vi "Vizualise Filter.vi"(10 "Reference Signal":waveform(dbl), 11 "CtlRef":refnum<vi>) -> (0 "Order":i32, 1 "Fc Low":dbl, 2 "Fc High":dbl, 3 "Type":T1, 4 "Filter Magnitude":cluster{"f0":dbl, "df":dbl, "magnitude":dbl[]}(graph))   [LabVIEW 2014]
uses:
  <vilib>/Analysis/3filter.llb/Filter Passband Type.ctl
  <vilib>/Utility/miscctls.llb/LVOutOfRangeActionTypeDef.ctl
  <vilib>/Analysis/3filter.llb/Butterworth Filter (DBL).vi
  <vilib>/express/express analysis/Spectral/Block/exnSpectralBlock spectral measurements peak poly.vi
  <vilib>/express/express analysis/Spectral/Block/exnSpectralBlock spectral measurements peak WFM.vi
  <vilib>/express/express analysis/Spectral/XNode/ExpressSpectralMeasurementsBlockNode.xnode
  <vilib>/Analysis/NI_AALBase.lvlib
  <vilib>/measure/NI_MABase.lvlib
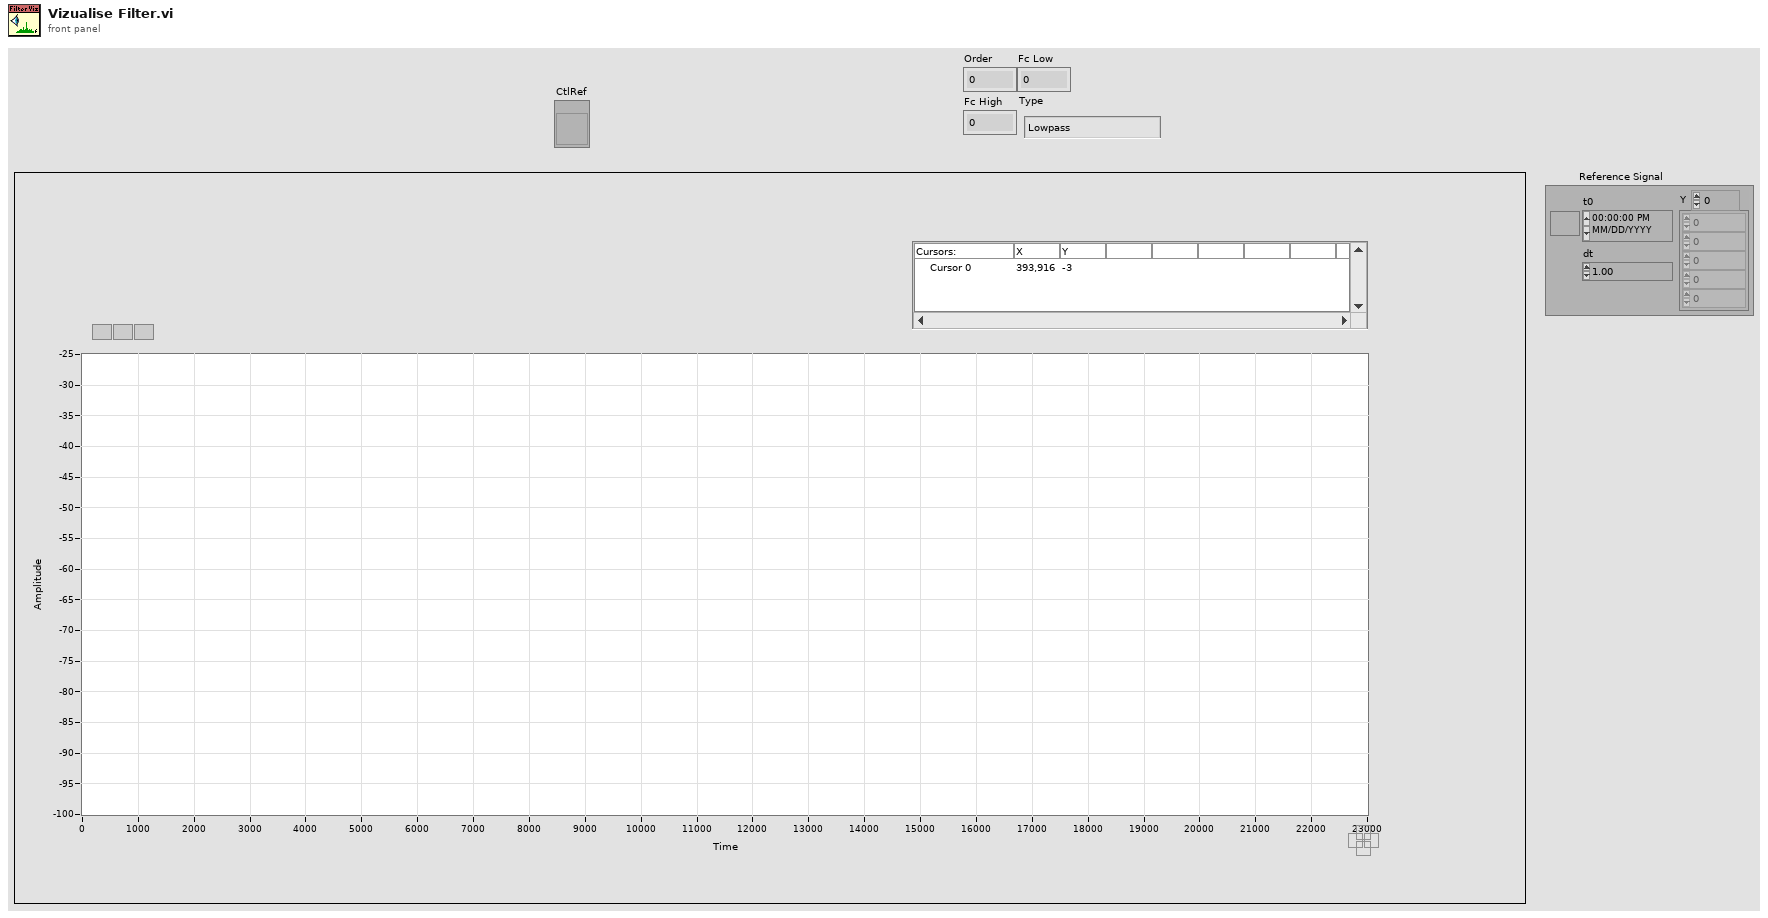
[diagram p1: front panel]
types:
  T1 = typedef "NI_AALBase.lvlib/Filter Passband Type.ctl" = enum32{"Lowpass", "Highpass", "Bandpass", "Bandstop"}
  T2 = typedef "LVOutOfRangeActionTypeDef.ctl" = cluster{"Out of Range Action Minimum":u8, "Out of Range Action Maximum":u8, "Out of Range Action Increment":u8}
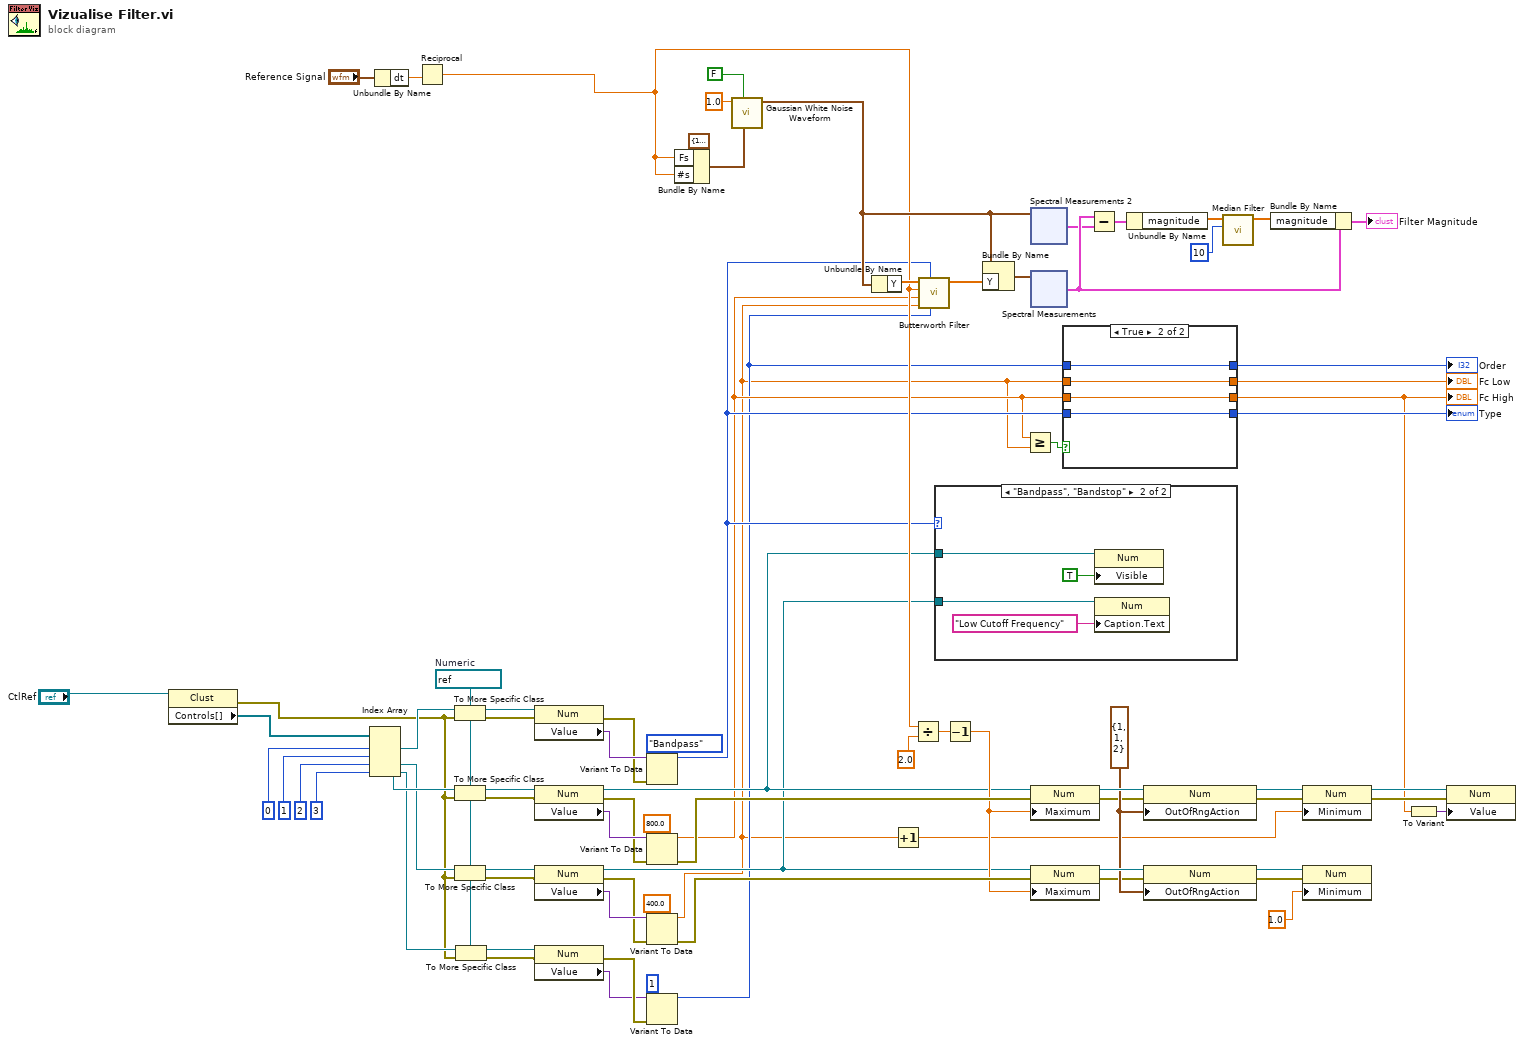
[diagram p0: block diagram]
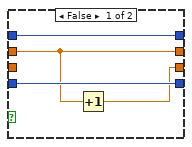
[diagram p2: hidden frame]
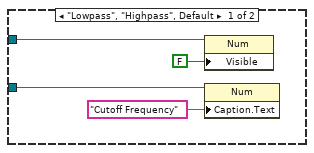
[diagram p3: hidden frame]
diagram:
  w46 = T2 {"Out of Range Action Minimum"=1, "Out of Range Action Maximum"=1, "Out of Range Action Increment"=2} ("Response to Value Outside Limits")
  w51 = refnum<vi> refnum  # Numeric
  n1 = property class="Clust"(reference="CtlRef") -> (error out=w24:errorcluster, "Controls[]"=w65:refnum<vi>[])  [unwired: 1 in, 1 out]
  n2 = Index Array(array=w65, index #1=0 ("index"), index #2=1 ("index"), index #3=2 ("index"), index #4=3 ("index")) -> (element #1=w60:refnum<vi>, element #2=w59:refnum<vi>, element #3=w58:refnum<vi>, element #4=w57:refnum<vi>)
  n3 = Unbundle By Name("Reference Signal") -> ("dt"=w17:dbl)
  n4 = Reciprocal(x=w17) -> (1/x=w16:dbl)
  n5 = To More Specific Class(target class=w51, reference=w60, error in=w24) -> (specific class reference=w56:refnum<vi>, error out=w55:errorcluster)
  n6 = To More Specific Class(target class=w51, reference=w59, error in=w24) -> (specific class reference=w34:refnum<vi>, error out=w35:errorcluster)
  n7 = To More Specific Class(target class=w51, reference=w58, error in=w24) -> (specific class reference=w33:refnum<vi>, error out=w36:errorcluster)
  n8 = To More Specific Class(target class=w51, reference=w57, error in=w24) -> (specific class reference=w32:refnum<vi>, error out=w37:errorcluster)
  n9 = property class="Num"(reference=w56, error in=w55) -> (error out=w53:errorcluster, "Value"=w54:variant)  [unwired: 1 out]
  n10 = property class="Num"(reference=w34, error in=w35) -> (reference out=w15:refnum<vi>, error out=w28:errorcluster, "Value"=w41:variant)
  n11 = property class="Num"(reference=w33, error in=w36) -> (reference out=w14:refnum<vi>, error out=w27:errorcluster, "Value"=w40:variant)
  n12 = property class="Num"(reference=w32, error in=w37) -> (error out=w39:errorcluster, "Value"=w38:variant)  [unwired: 1 out]
  n13 = Variant To Data(error in=w53, type=Filter_Passband_Type."Bandpass" ("filter type"), Variant=w54) -> (data=w11:T1)  [unwired: 1 out]
  n14 = Variant To Data(error in=w28, type=800.0 ("high cutoff freq"), Variant=w41) -> (data=w10:dbl, error out=w25:errorcluster)
  n15 = Variant To Data(error in=w27, type=400.0 ("low cutoff freq"), Variant=w40) -> (data=w1:dbl, error out=w26:errorcluster)
  n16 = Variant To Data(error in=w39, type=1 ("order"), Variant=w38) -> (data=w9:i32)  [unwired: 1 out]
  n17 = Bundle By Name(cluster=cluster{"Fs":dbl, "#s":dbl} {"Fs"=10000.0, "#s"=10000.0} ("sampling info"), "Fs"=w16, "#s"=w16) -> (w76:cluster{"Fs":dbl, "#s":dbl})
  n18 = call <vilib>:"Gaussian White Noise Waveform.vi"("sampling info"=w76, "reset signal"=FALSE, "standard deviation"=1.0 ("amplitude")) -> ("signal out"=w23:waveform(dbl))  [unwired: 7 in, 1 out]
  n19 = Unbundle By Name(w23) -> ("Y"=w78:dbl[])
  n20 = Increment(x=w1) -> (x+1=w13:dbl)
  n21 = Divide(x=w16, y=2.0) -> (x/y=w22:dbl)
  n22 = call-poly <vilib>:"Butterworth Filter.vi"("order"=w9, "filter type"=w11, "low cutoff freq: fl"=w1, "high cutoff freq: fh"=w10, "sampling freq: fs"=w16, "X"=w78) -> ("Filtered X"=w80:dbl[])  [unwired: 2 in, 1 out]
  n23 = case shown="\"Bandpass\", \"Bandstop\"" w11 {
    tunnel: w15 -> [w82 w86]
    tunnel: w14 -> [w81 w85]
    frame "Lowpass", "Highpass", Default {
      n24 = property class="Num"(reference=w82, "Visible"=FALSE) -> ()  [unwired: 1 in, 2 out]
      n25 = property class="Num"(reference=w81, "Caption.Text"="Cutoff Frequency") -> ()  [unwired: 1 in, 2 out]
    }
    frame "Bandpass", "Bandstop" {
      n26 = property class="Num"(reference=w86, "Visible"=TRUE) -> ()  [unwired: 1 in, 2 out]
      n27 = property class="Num"(reference=w85, "Caption.Text"="Low Cutoff Frequency") -> ()  [unwired: 1 in, 2 out]
    }
  }
  n28 = Decrement(x=w22) -> (x-1=w20:dbl)
  n29 = Bundle By Name(cluster=w23, "Y"=w80) -> (w68:waveform(dbl))
  n30 = Greater Or Equal?(x=w10, y=w1) -> (x >= y?=w12:bool)
  n31 = xnode ("Spectral Measurements 2")("Signals"=w23) -> ("FFT - (Peak)"=w67:cluster{"f0":dbl, "df":dbl, "magnitude":dbl[]})  [unwired: 1 in, 2 out]
  n32 = xnode ("Spectral Measurements")("Signals"=w68) -> ("FFT - (Peak)"=w71:cluster{"f0":dbl, "df":dbl, "magnitude":dbl[]})  [unwired: 1 in, 2 out]
  n33 = property class="Num"(reference=w15, error in=w25, "Maximum"=w20) -> (reference out=w50:refnum<vi>, error out=w45:errorcluster)
  n34 = property class="Num"(reference=w14, error in=w26, "Maximum"=w20) -> (reference out=w49:refnum<vi>, error out=w44:errorcluster)
  n35 = case shown="True" w12 {
    tunnel: w11 -> [w92 w93]
    tunnel: w10 -> [_ w94]
    tunnel: w1 -> [w90 w95]
    tunnel: w9 -> [w91 w96]
    tunnel: [w92 w93] -> w8
    tunnel: [w89 w94] -> w3
    tunnel: [w90 w95] -> w7
    tunnel: [w91 w96] -> w6
    frame False {
      n36 = Increment(x=w90) -> (x+1=w89:dbl)
    }
    frame True {
    }
  }
  "Order" <- w6
  "Fc Low" <- w7
  "Fc High" <- w3
  "Type" <- w8
  n37 = Subtract(x=w71, y=w67) -> (x-y=w74:cluster{"f0":dbl, "df":dbl, "magnitude":dbl[]})
  n38 = Unbundle By Name(w74) -> ("magnitude"=w73:dbl[])
  n39 = property class="Num"(reference=w50, error in=w45, "OutOfRngAction"=w46) -> (reference out=w48:refnum<vi>, error out=w42:errorcluster)
  n40 = property class="Num"(reference=w49, error in=w44, "OutOfRngAction"=w46) -> (reference out=w47:refnum<vi>, error out=w43:errorcluster)
  n41 = call <vilib>:"Median Filter.vi"("left rank"=10, "X"=w73) -> ("Filtered X"=w70:dbl[])  [unwired: 8 in, 1 out]
  n42 = Bundle By Name(cluster=w71, "magnitude"=w70) -> (→"Filter Magnitude":cluster{"f0":dbl, "df":dbl, "magnitude":dbl[]})
  n43 = property class="Num"(reference=w48, error in=w42, "Minimum"=w13) -> (reference out=w5:refnum<vi>, error out=w4:errorcluster)
  n44 = property class="Num"(reference=w47, error in=w43, "Minimum"=1.0 ("Data Entry Limits:Minimum")) -> ()  [unwired: 2 out]
  n45 = To Variant(anything=w3) -> (Variant=w2:variant)
  n46 = property class="Num"(reference=w5, error in=w4, "Value"=w2) -> ()  [unwired: 2 out]
